vi "fftw_malloc.vi"(8 "error in (no error)":errorcluster, 11 "bytes count":u32=256) -> (0 "error out":errorcluster, 3 "*data":u64)   [LabVIEW 2020, in "FFTWDLL.lvlib"]
doc: "Allocate FFTW memory aligned for SIMD."
uses:
  FFTWDLL.lvlib
  dll/libfftw3-3.dll
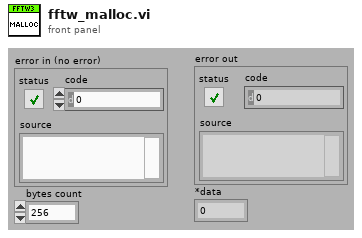
[diagram p1: front panel]
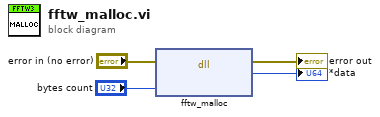
[diagram p0: block diagram]
diagram:
  n1 = dll-call lib="F:/FFTWDLL/dll/libfftw3-3.dll" fn="fftw_malloc"(error in="error in (no error)", "n"="bytes count") -> (error out=→"error out":errorcluster, "return type"=→"*data":u64)  [unwired: 3 in, 1 out]
